vi "FTW-Test-Subscriber-Disconnected.vi"() -> ()   [LabVIEW 2013]
uses:
  source/actor/Subscriber/FTW-Subscriber.lvclass
  source/actor/Ether/FTW-Ether.lvclass
panel:
  in  "Wait Time (ms)":u32=1000
  out "Results":T1(array[cluster])
  in  "Addresses":string[](array[string])=["inproc://*", "tcp://127.0.0.1/*"]
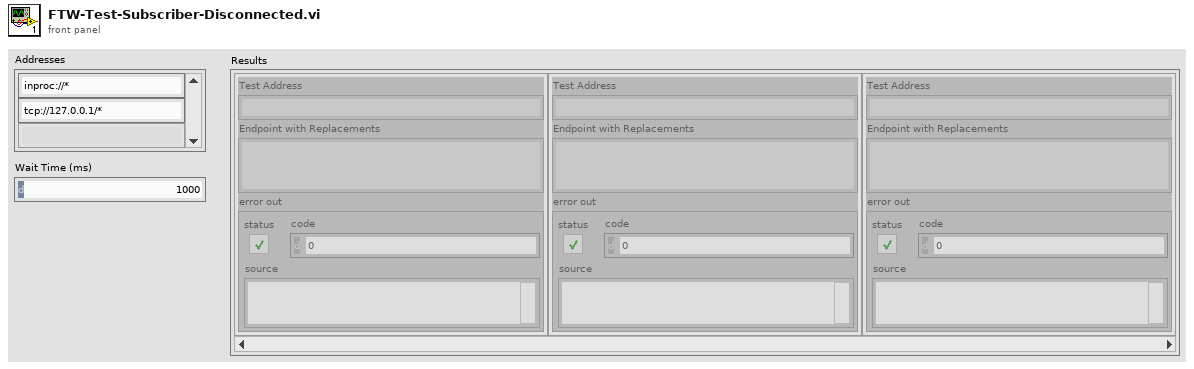
[diagram p1: front panel]
types:
  T1 = cluster{"Test Address":string, "Endpoint with Replacements":string, "error out":errorcluster}[]
  T2 = cluster{"String":string, "Endpoint with Replacements":string, "error out":errorcluster}
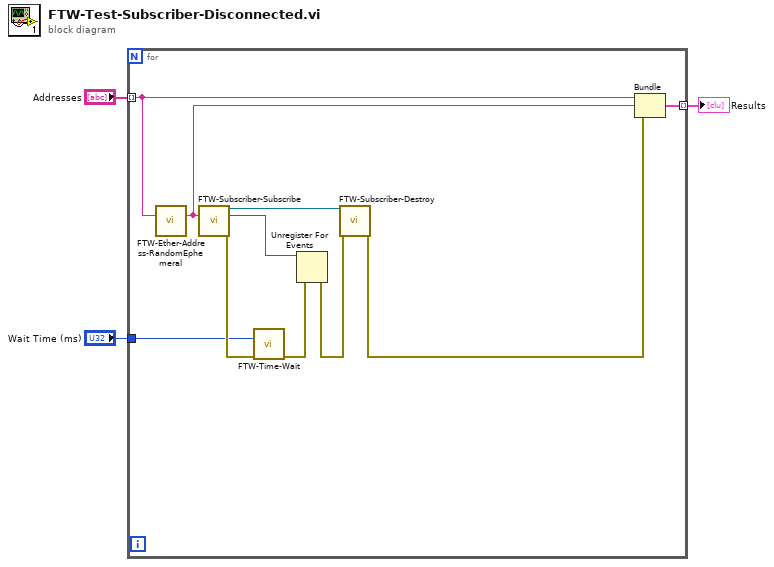
[diagram p0: block diagram]
diagram:
  n1 = for {
    tunnel: "Addresses" -> [w7] mode=indexing
    tunnel: [w5] -> w2 mode=indexing
    tunnel: "Wait Time (ms)" -> [w4]
    n2 = call "FTW-Ether-Address-RandomEphemeral.vi"("Endpoint"=w7) -> ("Endpoint with Replacements"=w8:string)  [unwired: 13 in, 1 out]
    n3 = call "FTW-Subscriber-Subscribe.vi"("Addresses"=w8) -> ("FTW-Subscription Out"=w9:refnum<class "FTW-Subscriber.lvclass">, "Subscriber Registration"=w10:refnum<event-registration>, "error out"=w13:errorcluster)  [unwired: 12 in]
    n4 = call "FTW-Time-Wait.vi"("Wait Time (ms)"=w4, "error in"=w13) -> ("error out"=w12:errorcluster)  [unwired: 13 in]
    n5 = Unregister For Events(event registration refnum=w10, error in=w12) -> (error out=w11:errorcluster)
    n6 = call "FTW-Subscriber-Destroy.vi"("FTW-Subscription In"=w9, "error in"=w11) -> ("error out"=w6:errorcluster)  [unwired: 13 in]
    n7 = Bundle("String"=w7, "Endpoint with Replacements"=w8, "error out"=w6) -> (w5:T2)  [unwired: 1 in]
  }
  "Results" <- w2
